vi "TestConvertToNamepath.vi"() -> ()   [LabVIEW 2017]
uses:
  Mapper/ExposeObjectMapNamepathData.ctl
  Mapper/ExposeMapperDataTypeEnum.ctl
  Mapper/ExposeObjectMapContainerTypeEnum.ctl
panel:
  out "Array":T1[](array[typedef])
  in  "StreamConfig":T4={"ClockRate"=4000.0, "UpdateTime"=50.0, "IntegrationTime"=1.0, "CollectionWindow"=5000.0, "PadWithZeros"=TRUE, "AutoAdjustRates"=TRUE} caption="Stream Device Config" {"UpdateTime" min=5.0 max=3000.0 step=1.0}
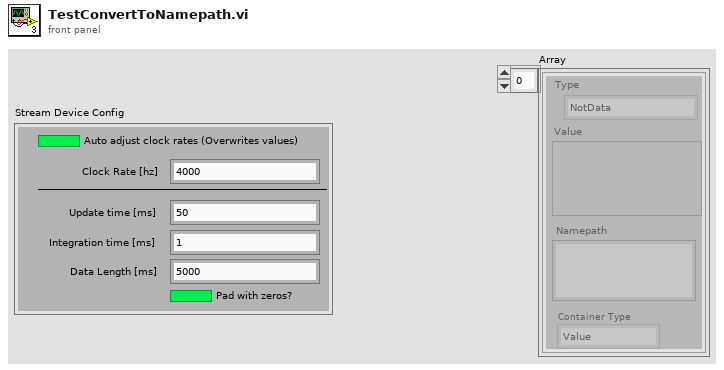
[diagram p1: front panel]
types:
  T1 = typedef "ExposeObjectMapNamepathData.ctl" = cluster{"Type":T2, "Value":variant, "Namepath":string, "Container Type":T3}
  T2 = typedef "ExposeMapperDataTypeEnum.ctl" = enum16{"NotData", "int8", "byte", "int16", "uint16", "int32", "uint32", "int64", "uint64", "Single", "Double", "String", "Boolean", "Container"}
  T3 = typedef "ExposeObjectMapContainerTypeEnum.ctl" = enum16{"Value", "Array", "Waveform", "NetContainer"}
  T4 = cluster{"ClockRate":dbl, "UpdateTime":dbl, "IntegrationTime":dbl, "CollectionWindow":dbl, "PadWithZeros":bool, "AutoAdjustRates":bool}
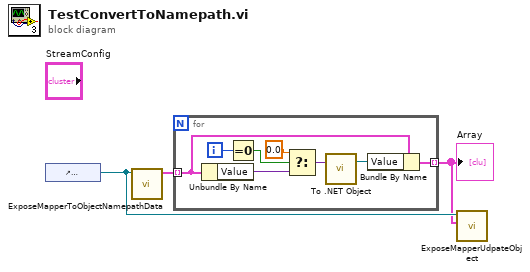
[diagram p0: block diagram]
diagram:
  n1 = control-ref of="StreamConfig"() -> (w3:refnum<vi>)
  n2 = call "ExposeMapperToObjectNamepathData.vi"("Value"=w3) -> ("Object map"=w2:T1[])  [unwired: 10 in]
  n3 = for {
    tunnel: w2 -> [w11] mode=indexing
    tunnel: [w9] -> w1 mode=indexing
    i -> [w4]
    n4 = Unbundle By Name(w11) -> ("Value"=w6:variant)
    n5 = Equal To 0?(x=w4) -> (x = 0?=w8:bool)
    n6 = Select(t=0.0, s=w8, f=w6) -> (s? t:f=w5:variant)
    n7 = call <vilib>:"To .NET Object.vi"("anything"=w5) -> (".NET object"=w10:refnum<k24>)  [unwired: 1 in, 1 out]
    n8 = Bundle By Name(cluster=w11, "Value"=w10) -> (w9:T1)
  }
  "Array" <- w1
  n9 = call "ExposeMapperUdpateObject.vi"("Object Map"=w1, "Type (or value to update)"=w3) -> ()  [unwired: 8 in, 2 out]
